vi "$IO_18v7Open.vi"(6 "error in":errorcluster={"status"=TRUE, "code"=-1073807346, "source"="VISA Write in IO_18v7Open.vi"}, 10 "Pump Control Ref.Sim":refnum<vi>, 11 "Runtime VISA name":refnum<visa-resource-name>="COM5") -> (2 "Connected":bool, 3 "VISA Refnum out":refnum<visa-resource-name>, 4 "error out":errorcluster={"status"=TRUE, "code"=-1073807346, "source"="VISA Write in IO_18v7Open.vi"})   [LabVIEW 2024]
uses:
  <vilib>/Instr/_visa.llb/VISA Configure Serial Port (Instr).vi
panel:
  out "ComPort Active":refnum<visa-resource-name>
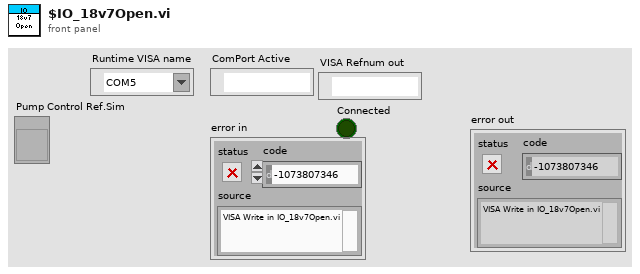
[diagram p1: front panel]
types:
  T1 = enum32{"invalid app kind", "Development System", "Run Time System", "Student Edition", "Embedded LabVIEW", "Evaluation", "Custom"}
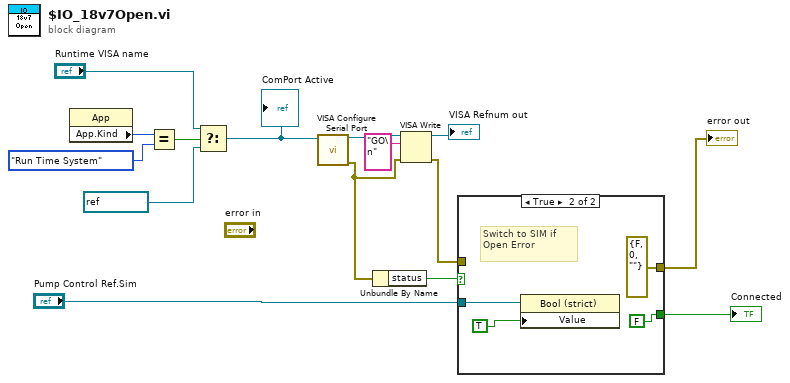
[diagram p0: block diagram]
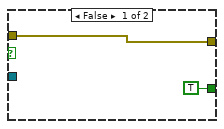
[diagram p2: hidden frame]
diagram:
  n1 = property class="App"() -> ("App.Kind"=w12:T1)  [unwired: 2 in, 2 out]
  n2 = Equal?(x=w12, y=T1."Run Time System") -> (x = y?=w10:bool)
  n3 = Select(t="Runtime VISA name", s=w10, f=refnum<visa-resource-name> "COM5" ("VISA resource name")) -> (s? t:f=w7:refnum<visa-resource-name>)
  "ComPort Active" <- w7
  n4 = call-poly "VISA Configure Serial Port"("VISA resource name"=w7) -> ("VISA resource name out"=w13:refnum<visa-resource-name>, "error out"=w3:errorcluster)  [unwired: 13 in]
  n5 = Unbundle By Name(w3) -> ("status"=w1:bool)
  n6 = VISA Write(VISA resource name=w13, write buffer="GO\n", error in (no error)=w3) -> (VISA resource name out=→"VISA Refnum out":refnum<visa-resource-name>, error out=w6:errorcluster)  [unwired: 1 out]
  n7 = case shown="True" w1 {
    tunnel: w6 -> [w17 _]
    tunnel: [w17 errorcluster {"status"=FALSE, "code"=0, "source"=""} ("error out")] -> w5
    tunnel: "Pump Control Ref.Sim" -> [_ w21]
    tunnel: [TRUE FALSE] -> w2
    frame False {
    }
    frame True {
      # "Switch to SIM if \nOpen Error"
      n8 = property class="Bool (strict)"(reference=w21, "Value"=TRUE) -> ()  [unwired: 1 in, 2 out]
    }
  }
  "error out" <- w5
  "Connected" <- w2
